vi "RunTestCalled.vi"(1 "TestCaseMock In":refnum<class "TestCaseMock.lvclass">) -> (0 "RunTest Called":bool)   [LabVIEW 2019, in "TestResultTest.lvlib" / "Support.lvlib" / "TestCaseMock.lvclass"]
uses:
  TestCaseMock.lvclass
  TestCaseMock.lvclass/TestCaseMock.ctl
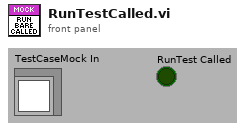
[diagram p1: front panel]
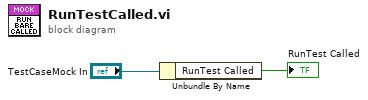
[diagram p0: block diagram]
diagram:
  n1 = Unbundle By Name("TestCaseMock In") -> ("RunTest Called"=→"RunTest Called":bool)
